vi "Experiment-2-5-2.vi"() -> ()   [LabVIEW 2014]
panel:
  in  "Offset":dbl
  in  "stop":bool
  in  "Frequency":dbl
  in  "Amplitude":dbl
  out "Waveform Chart":dbl(graph)
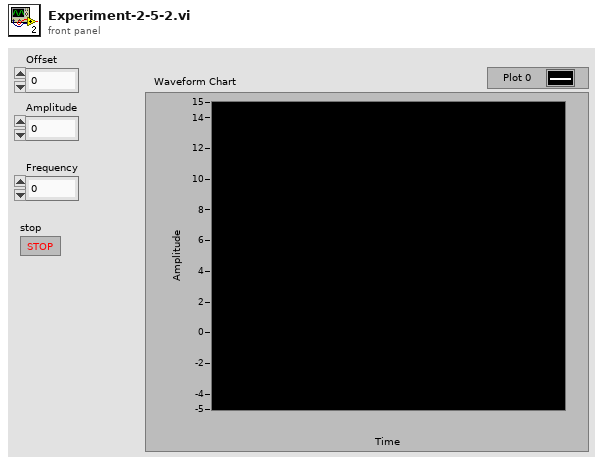
[diagram p1: front panel]
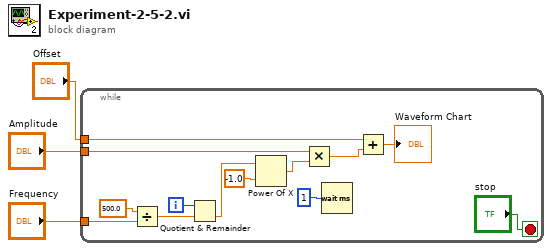
[diagram p0: block diagram]
diagram:
  n1 = while {
    tunnel: "Frequency" -> [w11]
    tunnel: "Amplitude" -> [w7]
    tunnel: "Offset" -> [w4]
    i -> [w14]
    stop <- "stop" stop-if-true
    n2 = Divide(x=500.0, y=w11) -> (x/y=w13:dbl)
    n3 = Quotient & Remainder(x=w14, y=w13) -> (floor(x/y)=w9:dbl)  [unwired: 1 out]
    n4 = Power Of X(1:-1.0, 2:w9) -> (0:w8:dbl)
    n5 = Multiply(x=w7, y=w8) -> (x*y=w6:dbl)
    n6 = Wait (ms)(milliseconds to wait=1) -> ()  [unwired: 1 out]
    n7 = Add(x=w4, y=w6) -> (x+y=→"Waveform Chart":dbl)
  }
